vi "recursively populate local tree ctl.vi"(8 "error in (no error)":errorcluster, 10 "Object path":string="IndivITX/Test1/SA03008N.20190801.000000.itx", 11 "tree ctl ref":refnum<vi>) -> (0 "error out":errorcluster, 3 "reference out":refnum<vi>)   [LabVIEW 2016]
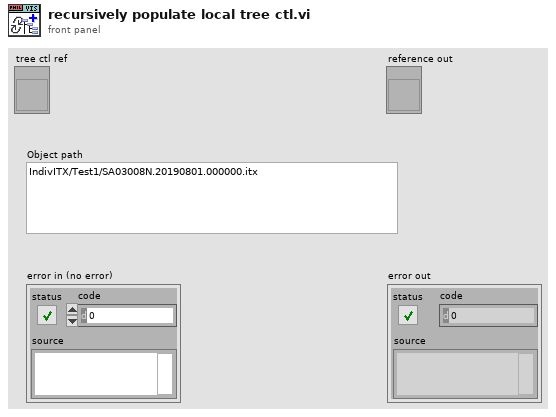
[diagram p1: front panel]
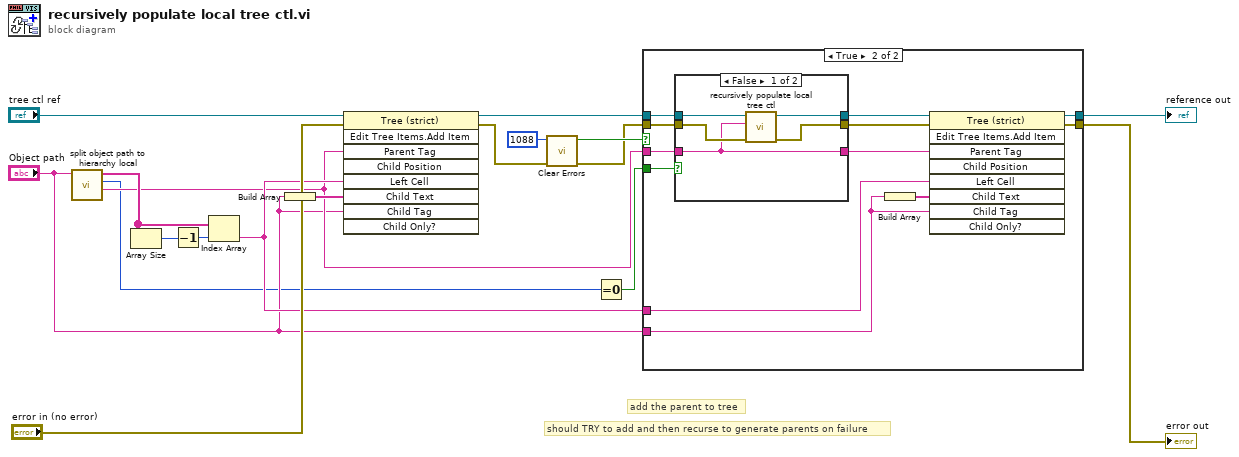
[diagram p0: block diagram]
diagram:
  # "should TRY to add and then recurse to generate parents on failure"
  # "add the parent to tree"
  n1 = call "split object path to hierarchy local.vi"("Object path"="Object path") -> ("parent path"=w4:string, "layers"=w2:i32, "hierarchy"=w7:string[])  [unwired: 8 in]
  n2 = Array Size(array=w7) -> (size(s)=w6:i32)
  n3 = Decrement(x=w6) -> (x-1=w9:i32)
  n4 = Index Array(array=w7, index=w9) -> (element=w5:string)
  n5 = Build Array("Object path") -> (w16:string[])
  n6 = invoke on="Invoke Node" class="Tree (strict)" method="Edit Tree Items.Add Item"(reference="tree ctl ref", error in="error in (no error)", "Parent Tag"=w4, "Left Cell"=w5, "Child Text"=w16, "Child Tag"="Object path") -> (reference out=w14:refnum<vi>, error out=w1:errorcluster)  [unwired: 3 in, 7 out]
  n7 = call <vilib>:"Clear Errors.vi"("error in (no error)"=w1, "specific error code to clear (0: all)"=1088) -> ("error out"=w8:errorcluster, "specific error cleared?"=w13:bool)  [unwired: 4 in]
  n8 = Equal To 0?(x=w2) -> (x = 0?=w18:bool)
  n9 = case shown="True" w13 {
    tunnel: [w19 w27] -> w11
    tunnel: w18 -> [_ w32]
    tunnel: [w20 w28] -> w10
    tunnel: w8 -> [w19 w22]
    tunnel: w4 -> [_ w31]
    tunnel: w14 -> [w20 w23]
    tunnel: "Object path" -> [_ w21]
    tunnel: w5 -> [_ w24]
    frame False {
    }
    frame True {
      n10 = case shown="False" w32 {
        tunnel: w22 -> [w37 w40]
        tunnel: w31 -> [w33 w38]
        tunnel: [w36 w40] -> w30
        tunnel: w23 -> [w35 w39]
        tunnel: [w34 w39] -> w29
        tunnel: [w33 w38] -> w26
        frame False {
          n11 = call "recursively populate local tree ctl.vi"("error in (no error)"=w37, "Object path"=w33, "tree ctl ref"=w35) -> ("error out"=w36:errorcluster, "reference out"=w34:refnum<vi>)  [unwired: 7 in]
        }
        frame True {
        }
      }
      n12 = Build Array(w21) -> (w25:string[])
      n13 = invoke on="Invoke Node" class="Tree (strict)" method="Edit Tree Items.Add Item"(reference=w29, error in=w30, "Parent Tag"=w26, "Left Cell"=w24, "Child Text"=w25, "Child Tag"=w21) -> (reference out=w28:refnum<vi>, error out=w27:errorcluster)  [unwired: 3 in, 7 out]
    }
  }
  "error out" <- w11
  "reference out" <- w10
